vi "Read.vi"(8 "error in (no error)":errorcluster, 11 "Time Stamp Array in":refnum<class "Time Stamp Array.lvclass">) -> (0 "error out":errorcluster, 2 "String Array":timestamp[](array[timestamp]), 3 "Time Stamp Array out":refnum<class "Time Stamp Array.lvclass">)   [LabVIEW 2020, in "Data.lvlib" / "Time Stamp Array.lvclass"]
doc: "Read Time Stamp Array."
uses:
  Time Stamp Array.lvclass
  Time Stamp Array.lvclass/Time Stamp Array.ctl
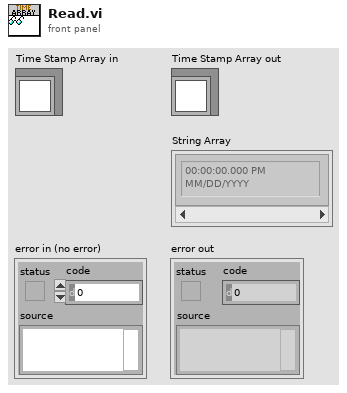
[diagram p1: front panel]
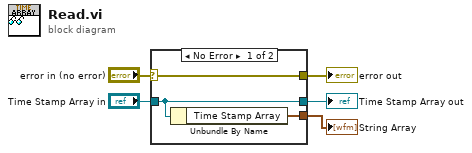
[diagram p0: block diagram]
diagram:
  n1 = case shown="No Error" "error in (no error)" {
    selector: "error in (no error)" -> [w8 w9]
    tunnel: [w8 w9] -> w4
    tunnel: [w7 w10] -> w2
    tunnel: "Time Stamp Array in" -> [w7 w10]
    tunnel: [w6 _] -> w1
    frame No Error {
      n2 = Unbundle By Name(w7) -> ("Time Stamp Array"=w6:timestamp[])
    }
    frame Error {
    }
  }
  "error out" <- w4
  "Time Stamp Array out" <- w2
  "String Array" <- w1
